vi "Set DAQ Offset.vi"(8 "error in (no error)":errorcluster, 10 "Offsets":dbl[](array[numeric]), 11 "Instrument.DAQ":refnum<class "Instrument.DAQ.lvclass">) -> (0 "error out":errorcluster, 3 "Instrument.DAQ out":refnum<class "Instrument.DAQ.lvclass">)   [LabVIEW 2019, in "Instrument.DAQ.lvclass"]
uses:
  Instrument.DAQ.lvclass
  Instrument.DAQ.lvclass/Instrument.DAQ.ctl
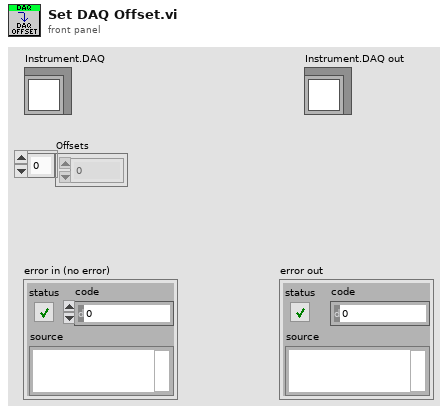
[diagram p1: front panel]
types:
  T1 = typedef "Instrument.DAQ.lvclass/Channel.Gain--Cluster--Array.ctl" = T2[]
  T2 = typedef "Instrument.DAQ.lvclass/Channel.Gain--Cluster.ctl" = cluster{"Channel":string, "Gain":dbl}
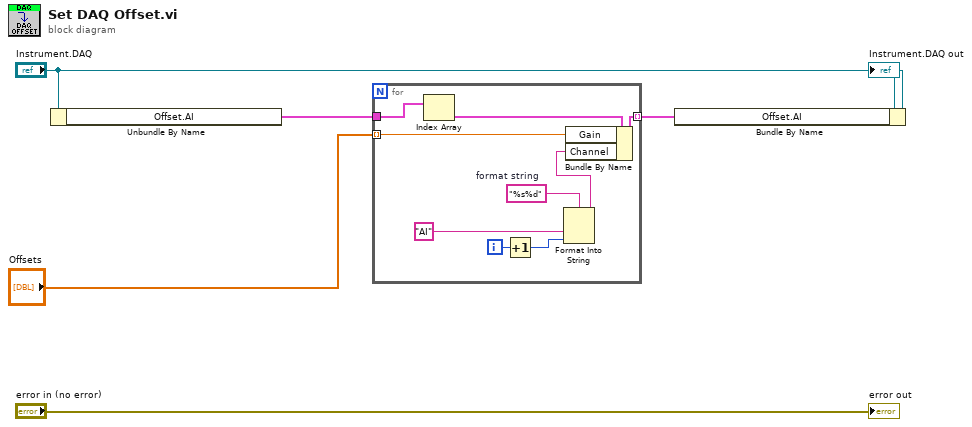
[diagram p0: block diagram]
diagram:
  n1 = Unbundle By Name("Instrument.DAQ") -> ("Offset.AI"=w6:T1)
  n2 = for {
    tunnel: w6 -> [w15]
    tunnel: [w14] -> w2 mode=indexing
    tunnel: "Offsets" -> [w9] mode=indexing
    i -> [w13]
    w12 = "%s%d"  # format string
    n3 = Index Array(array=w15) -> (element=w8:T2)  [unwired: 1 in]
    n4 = Increment(x=w13) -> (x+1=w10:i32)
    n5 = Format Into String(format string=w12, "AI" ("input 1"), w10) -> (resulting string=w11:string)  [unwired: 2 in, 1 out]
    n6 = Bundle By Name(cluster=w8, "Gain"=w9, "Channel"=w11) -> (w14:T2)
  }
  n7 = Bundle By Name(cluster="Instrument.DAQ", "Offset.AI"=w2) -> (→"Instrument.DAQ out":refnum<class "Instrument.DAQ.lvclass">)
  "error out" <- "error in (no error)"
